vi "workspace.from_rid.vi"(8 "error in":errorcluster, 10 "Workspace RID":string, 11 "Nominal Client in":refnum<class "Nominal Client.lvclass">) -> (0 "error out":errorcluster, 2 "Workspace":refnum<class "workspace.lvclass">, 3 "Nominal Client out":refnum<class "Nominal Client.lvclass">)   [LabVIEW 2020, in "Nominal Client.lvclass"]
doc: "Gets the workspace with the specified WorkspaceRid."
uses:
  Nominal Client.lvclass
  nominal types/workspace/workspace.lvclass
  Nominal Client.lvclass/Nominal Client.ctl
  create.authorization_header.vi
  trace.payload_sent.vi
  trace.payload_received.vi
  error.vi
  api_token.get.vi
  error.vi/859f8e04-e495-489b-b5b4-7ac163f56130.vi
  submodules/reqwest-labview/lv-src/reqwest/get.vi
  <vilib>/JDP Science/JSONtext/Get all Object Items.vi
  <vilib>/Utility/error.llb/Error Cluster From Error Code.vi
  <vilib>/JDP Science/JSONtext/JSON text to Variant.vi
  <vilib>/JDP Science/JSONtext/LVClass Serializer/JSONtext LVClass Serializer.lvclass
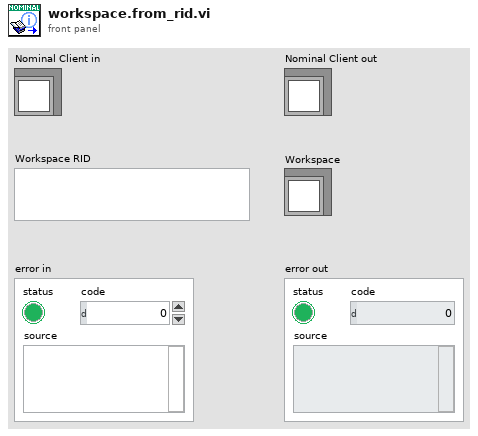
[diagram p1: front panel]
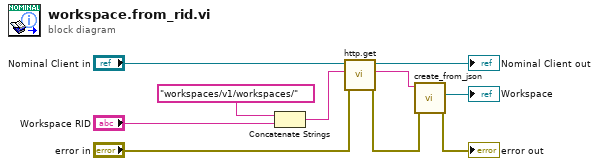
[diagram p0: block diagram]
diagram:
  n1 = Concatenate Strings("workspaces/v1/workspaces/" ("Path"), "Workspace RID") -> (w6:string)
  n2 = call "http.get.vi"("error in"="error in", "Path"=w6, "Nominal Client in"="Nominal Client in") -> ("error out"=w3:errorcluster, "Response"=w4:string, "Nominal Client out"=→"Nominal Client out":refnum<class "Nominal Client.lvclass">)  [unwired: 6 in]
  n3 = call "create_from_json.vi"("error in"=w3, "JSON"=w4) -> ("error out"=→"error out":errorcluster, "Workspace"=→"Workspace":refnum<class "workspace.lvclass">)  [unwired: 8 in]
